vi "Event Case to String.vi"(7 "Additional Info":string="Event Structure", 8 "error in (no error)":errorcluster, 10 "Type":T1, 11 "Control In":refnum<vi>) -> (0 "error out":errorcluster, 2 "Label.Text":string, 3 "Diagnostic String":string)   [LabVIEW 2017]
uses:
  <vilib>/event_ctls.llb/lveventtype.ctl
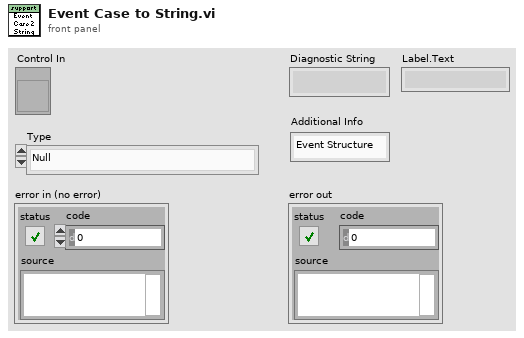
[diagram p1: front panel]
types:
  T1 = typedef "lveventtype.ctl" = enum32{"Null", "Timeout", "Annotation Menu Selection", "Annotation Menu Selection?", "App Instance Close", "App Instance Close?", "Autoscale Range Change", "Bookmark Info Change", "Cell Edit", "Cell Edit?", "Cursor Grab", "Cursor Grab?", "Cursor Menu Selection", "Cursor Menu Selection?", "Cursor Move", "Cursor Release", "Data Change", "Direction Change", "Display State Change", "Drag Ended", "Drag Enter", "Drag Leave", "Drag Over", "Drag Source Update", "Drag Starting", "Drag Starting?", "Drop", "Exec State Change", "Key Down", "Key Down?", "Key Repeat", "Key Repeat?", "Key Up", "Listbox Double Click", "Menu Activation?", "Menu Selection (App)", "Menu Selection? (App)", "Menu Selection (User)", "Mouse Down", "Mouse Down?", "Mouse Enter", "Mouse Leave", "Mouse Move", "Mouse Up", "Mouse Wheel", "NI Security User Change (App)", "Pane Size", "Panel Close", "Panel Close?", "Panel Resize", "Plot Attribute Change", "Scale Range Change", "Shortcut Menu Activation?", "Shortcut Menu Selection (App)", "Shortcut Menu Selection? (App)", "Shortcut Menu Selection (User)", "Tree Double Click", "Tree Drag", "Tree Drag?", "Tree Drop", "Tree Drop?", "Tree Item Close", "Tree Item Close?", "Tree Item Open", "Tree Item Open?", "User Event", "Value Change"}
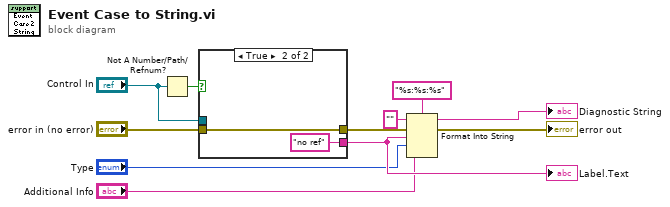
[diagram p0: block diagram]
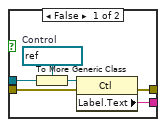
[diagram p2: hidden frame]
diagram:
  n1 = Not A Number/Path/Refnum?(number/path/refnum="Control In") -> (NaN/Path/Refnum?=w1:bool)
  n2 = case shown="True" w1 {
    tunnel: "error in (no error)" -> [w17 w19]
    tunnel: [w16 "no ref" ("Label.Text")] -> w8
    tunnel: [w15 w19] -> w4
    tunnel: "Control In" -> [w12 _]
    frame False {
      w14 = refnum<vi> refnum  # Control
      n3 = To More Generic Class(target class=w14, reference=w12) -> (generic class reference=w13:refnum<vi>)
      n4 = property class="Ctl"(reference=w13, error in=w17) -> (error out=w15:errorcluster, "Label.Text"=w16:string)  [unwired: 1 out]
    }
    frame True {
    }
  }
  "Label.Text" <- w8
  n5 = Format Into String(format string="%s:%s:%s", initial string="", error in=w4, w8, "Type", "Additional Info") -> (resulting string=→"Diagnostic String":string, error out=→"error out":errorcluster)
